vi "ukol2.vi"() -> ()   [LabVIEW 2023]
uses:
  <vilib>/addons/Digital Filter Design/Process.llb/DFD Filtering with State (Wfm).vi
  <vilib>/measure/NI_MABase.lvlib
  <vilib>/Analysis/NI_AALPro.lvlib
  <vilib>/addons/Digital Filter Design/NI_DigFilterLicensed.lvlib
panel:
  out "Homodynni detekce":waveform(dbl)[](graph)
  out "hilbert":waveform(dbl)[](graph)
  in  "amplitude":dbl=1.0 format="%0.2p"
  in  "frequency":dbl=10.0 format="%0.2p"
  out "Waveform Graph":waveform(dbl)[](graph)
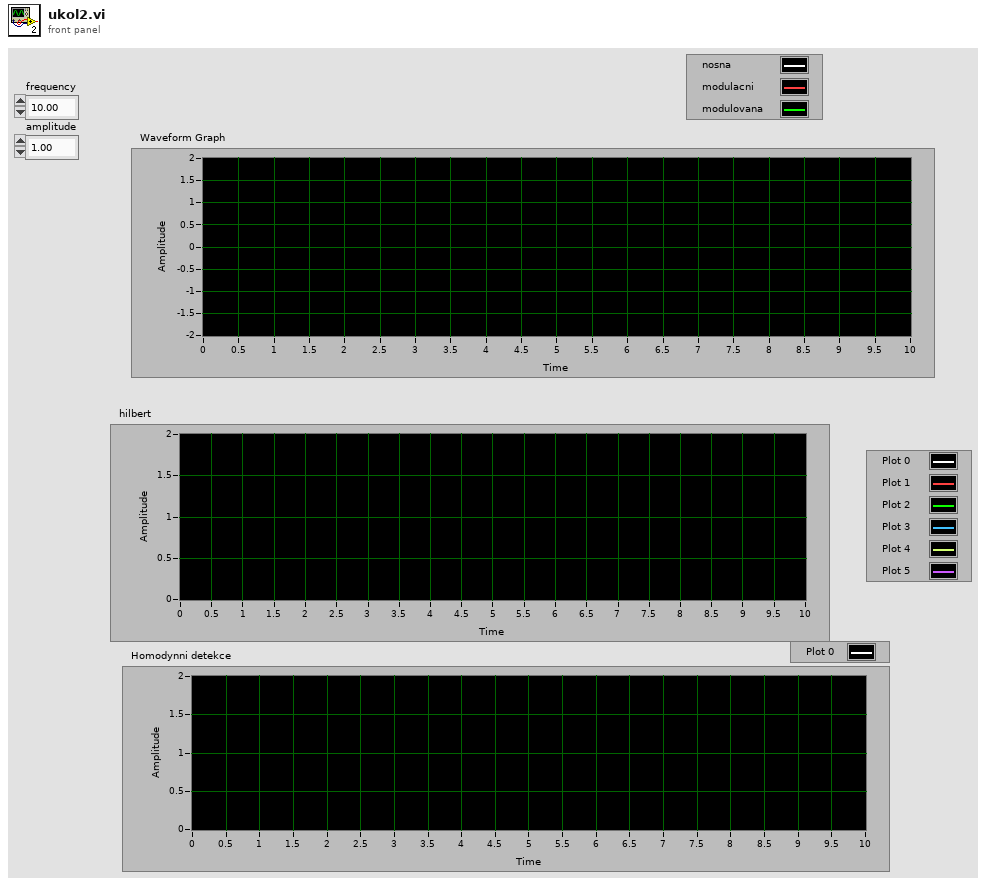
[diagram p1: front panel]
types:
  T1 = typedef "NI_DigFilterLicensed.lvlib/DFD Filter Obj.ctl" = cluster{"mSRate_Fs":dbl, "mSRate_Version":string, "mSRate_Comments":string, "mSRate_OrgCoef":T2, "mSRate_CurCoef":T2, "mSRate_Quantized?":bool, "mSRate_QCoef":T2, "mSRate_QSettings":T4[], "mSRate_Order":i32, "mSRate_Scaling":cluster{"mSRate_ScaleByPowerOf2?":bool, "mSRate_ScaleType":T6}}
  T2 = typedef "NI_DigFilterLicensed.lvlib/DFD Filter Coef.ctl" = cluster{"type":T3, "gain":dbl, "coef a (k)":dbl[], "coef b (v)":dbl[]}
  T3 = typedef "NI_DigFilterLicensed.lvlib/DFD Filter Structure Type Selector.ctl" = enum16{"Undefined", "FIR Direct Form", "FIR Direct Form Transposed", "FIR Symmetric", "FIR Antisymmetric", "IIR Direct Form I", "IIR Direct Form I Transposed", "IIR Direct Form II", "IIR Direct Form II Transposed", "IIR Cascaded Second Order Sections Form I", "IIR Cascaded Second Order Sections Form I Transposed", "IIR Cascaded Second Order Sections Form II", "IIR Cascaded Second Order Sections Form II Transposed", "Lattice Allpass (basic sections)", "Lattice Allpass (one multiplier sections)", "Lattice Allpass (normalized sections)", "Lattice AR (basic sections)", "Lattice AR (one multiplier sections)", "Lattice AR (normalized sections)", "Lattice MA (minimum phase)", "Lattice MA (maximum phase)", "Lattice ARMA (basic sections)", "Lattice ARMA (one multiplier sections)", "Lattice ARMA (normalized sections)"}
  T4 = typedef "NI_DigFilterLicensed.lvlib/dfd_Internal Quantization Settings.ctl" = cluster{"source":T5, "wl":i16, "iwl":i16, "overflow mode":enum16{"Saturation", "Wrap"}, "rounding mode":enum16{"Nearest", "Truncation"}, "signed?":bool}
  T5 = typedef "NI_DigFilterLicensed.lvlib/dfd_Internal Quantization Srcs.ctl" = u16
  T6 = typedef "NI_DigFilterLicensed.lvlib/DFD Coef Norm Type.ctl" = enum16{"No Norm", "Time Domain 1-Norm", "Time Domain 2-Norm", "Time Domain Inf-Norm"}
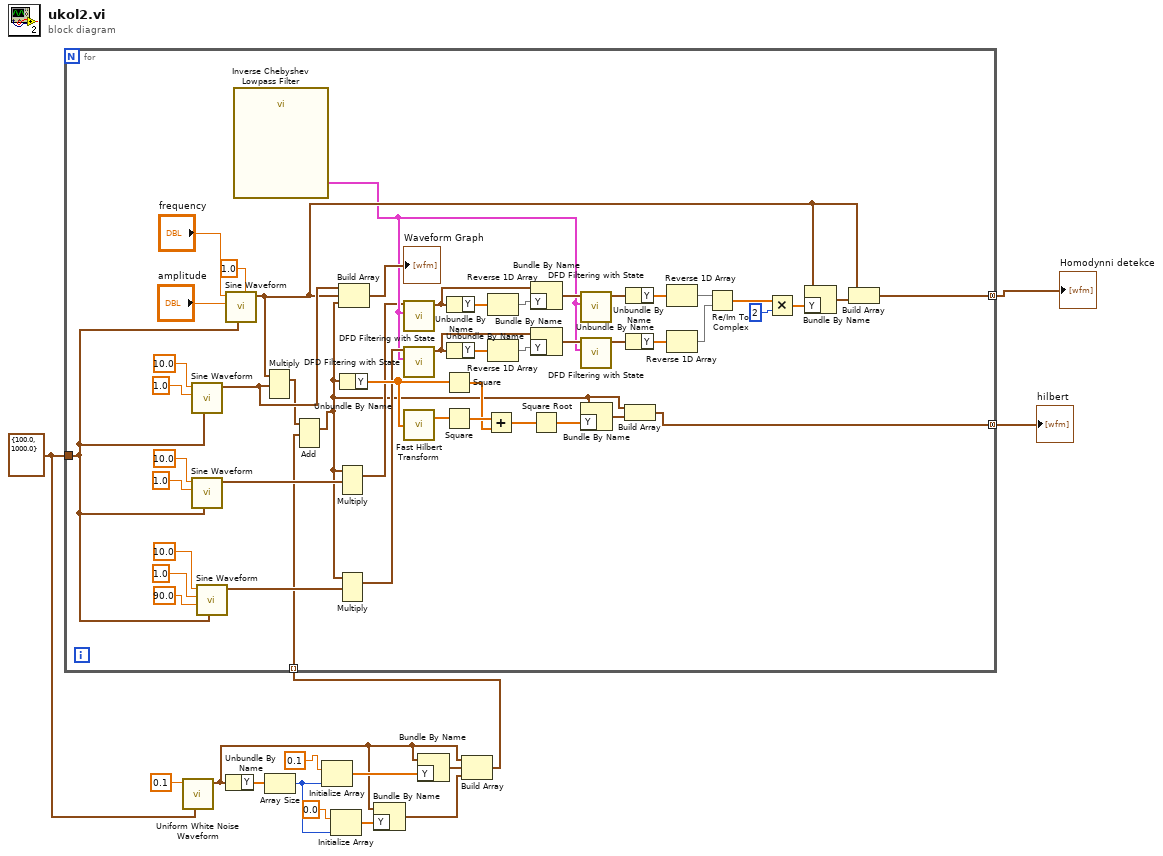
[diagram p0: block diagram]
diagram:
  w4 = cluster{"Fs":dbl, "#s":dbl} {"Fs"=100.0, "#s"=1000.0} ("sampling info")
  n1 = call <vilib>:"Uniform White Noise Waveform.vi"("sampling info"=w4, "amplitude"=0.1) -> ("signal out"=w6:waveform(dbl))  [unwired: 8 in, 1 out]
  n2 = Unbundle By Name(w6) -> ("Y"=w11:dbl[])
  n3 = Array Size(array=w11) -> (size(s)=w8:i32)
  n4 = Initialize Array(0.1 ("element"), w8) -> (w13:dbl[])
  n5 = Initialize Array(0.0 ("element"), w8) -> (w7:dbl[])
  n6 = Bundle By Name(cluster=w6, "Y"=w7) -> (w3:waveform(dbl))
  n7 = Bundle By Name(cluster=w6, "Y"=w13) -> (w10:waveform(dbl))
  n8 = Build Array(w6, w10, w3) -> (w5:waveform(dbl)[])
  n9 = for {
    tunnel: w5 -> [w19] mode=indexing
    tunnel: w4 -> [w18]
    tunnel: [w17] -> w1 mode=concatenating
    tunnel: [w16] -> w2 mode=concatenating
    n10 = call <vilib>:"Sine Waveform.vi"("sampling info"=w18, "amplitude"=1.0, "frequency"=10.0) -> ("signal out"=w60:waveform(dbl))  [unwired: 7 in, 1 out]
    n11 = call <vilib>:"Sine Waveform.vi"("sampling info"=w18, "amplitude"=1.0, "frequency"=10.0) -> ("signal out"=w47:waveform(dbl))  [unwired: 7 in, 1 out]
    n12 = call <vilib>:"Sine Waveform.vi"("sampling info"=w18, "phase"=90.0, "amplitude"=1.0, "frequency"=10.0) -> ("signal out"=w43:waveform(dbl))  [unwired: 6 in, 1 out]
    n13 = call <vilib>:"Sine Waveform.vi"("offset"=1.0, "sampling info"=w18, "amplitude"="amplitude", "frequency"="frequency") -> ("signal out"=w30:waveform(dbl))  [unwired: 6 in, 1 out]
    n14 = call "Inverse Chebyshev Lowpass Filter"() -> ("filter out"=w23:T1)  [unwired: 10 in, 1 out]
    n15 = Multiply(1:w60, 2:w30) -> (0:w20:waveform(dbl))  [unwired: 1 in, 1 out]
    n16 = Add(1:w19, 2:w20) -> (0:w15:waveform(dbl))  [unwired: 1 in, 1 out]
    n17 = Multiply(1:w47, 2:w15) -> (0:w22:waveform(dbl))  [unwired: 1 in, 1 out]
    n18 = Multiply(1:w43, 2:w15) -> (0:w38:waveform(dbl))  [unwired: 1 in, 1 out]
    n19 = Build Array(w60, w30, w15) -> (→"Waveform Graph":waveform(dbl)[])
    n20 = Unbundle By Name(w15) -> ("Y"=w55:dbl[])
    n21 = call-poly <vilib>:"DFD Filtering with State.vi"("filter"=w23, "signal in"=w22) -> ("signal out"=w27:waveform(dbl))  [unwired: 7 in, 2 out]
    n22 = call-poly <vilib>:"DFD Filtering with State.vi"("filter"=w23, "signal in"=w38) -> ("signal out"=w35:waveform(dbl))  [unwired: 7 in, 2 out]
    n23 = call <vilib>:"Fast Hilbert Transform.vi"("X"=w55) -> ("Hilbert{X}"=w56:dbl[])  [unwired: 1 out]
    n24 = Square(x=w55) -> (x^2=w53:dbl[])
    n25 = Square(x=w56) -> (x^2=w54:dbl[])
    n26 = Unbundle By Name(w27) -> ("Y"=w29:dbl[])
    n27 = Unbundle By Name(w35) -> ("Y"=w37:dbl[])
    n28 = Add(x=w54, y=w53) -> (x+y=w52:dbl[])
    n29 = Reverse 1D Array(array=w29) -> (reversed array=w28:dbl[])
    n30 = Reverse 1D Array(array=w37) -> (reversed array=w36:dbl[])
    n31 = Bundle By Name(cluster=w27, "Y"=w28) -> (w26:waveform(dbl))
    n32 = Bundle By Name(cluster=w35, "Y"=w36) -> (w34:waveform(dbl))
    n33 = Square Root(x=w52) -> (sqrt(x)=w51:dbl[])
    n34 = call-poly <vilib>:"DFD Filtering with State.vi"("filter"=w23, "signal in"=w26) -> ("signal out"=w24:waveform(dbl))  [unwired: 7 in, 2 out]
    n35 = call-poly <vilib>:"DFD Filtering with State.vi"("filter"=w23, "signal in"=w34) -> ("signal out"=w32:waveform(dbl))  [unwired: 7 in, 2 out]
    n36 = Bundle By Name(cluster=w15, "Y"=w51) -> (w50:waveform(dbl))
    n37 = Build Array(w15, w50) -> (w16:waveform(dbl)[])
    n38 = Unbundle By Name(w24) -> ("Y"=w25:dbl[])
    n39 = Unbundle By Name(w32) -> ("Y"=w33:dbl[])
    n40 = Reverse 1D Array(array=w25) -> (reversed array=w21:dbl[])
    n41 = Reverse 1D Array(array=w33) -> (reversed array=w31:dbl[])
    n42 = Re/Im To Complex(1:w31, 2:w21) -> (0:w42:cdb[])
    n43 = Multiply(x=w42, y=2) -> (x*y=w41:cdb[])
    n44 = Bundle By Name(cluster=w30, "Y"=w41) -> (w39:waveform(dbl))
    n45 = Build Array(w30, w39) -> (w17:waveform(dbl)[])
  }
  "Homodynni detekce" <- w1
  "hilbert" <- w2
